vi "DMM_Scan DER Configure and Measure.vi"(0 "Scan Resources Handles In":T2={"DMM Handle"="", "DAQmx Task Out"="", "Relays Status Array"=[], "N Shift Shunt"=1, "Close all Shunts?"=TRUE, "Relays Debounce Time (ms)"=5}, 5 "Scan Configuration":T3[](array[typedef]) {"Resolution in Digits" items=["3 1/2"=3.5, "4 1/2"=4.5, "5 1/2"=5.5, "6 1/2"=6.5, "7 1/2"=7.5]}, 11 "error in":errorcluster) -> (4 "Scan Resources Handles Out":T1={"DMM Handle"="", "DAQmx Task Out"="", "Relays Status Array"=[], "N Shift Shunt"=1, "Close all Shunts?"=TRUE, "Relays Debounce Time (ms)"=5}, 6 "Formatted Measurements":T6[](array[typedef]) {"Switch Time" format="%#_3p"}, 8 "Raw Measurements":T5[](array[typedef]) {"Value" format="%#_8g"}, 10 "Execution Settings":T7[](array[typedef]) {"Function" items=["DC Volts"=1, "AC Volts"=2, "DC Current"=3, "AC Current"=4, "2-Wire Resistance"=5, "4-Wire Resistance"=101, "Frequency"=104, "Period"=105, "AC Volts DC Coupled"=1001, "Diode"=1002, "Waveform Voltage"=1003, "Waveform Current"=1004, "Capacitance"=1005, "Inductance"=1006, "Temperature"=108]; "Absolute\nResolution" format="%#_6p"; "Input Resistance\n(Ohm)" format="%#_6p"; "Range" format="%#_6p"; "Minimum\nFrequency (Hz)" format="%#_6p"; "Aperture\nTime (s)" format="%#_6p"; "Auto Range\nValue" format="%#_6p"; "Settle\nTime (s)" format="%#_6p"}, 14 "Total Scan Time (s)":dbl format="%#.3p", 15 "error out":errorcluster)   [LabVIEW 2021, in "DMM_Scan DAQ Ext RLY.lvlib"]
doc: "Configures an NI-DMM Scan measurement list on the resource provided by the Scan Handle In control according to each given Channel, Function/Range, Digits sub-control. \n\nReturns Formatted Measurements based on Channels and Measurements (string with units), Out of Range, Measurement Time (including configuration, apperture and relay debounce).\n\nReturns Raw Measurements in numeric form to be used and compared in a sequencer.\n \nFor optimization, debugging and reporting, returns Execution Settings and Total Scan Time (s)"
uses:
  DMM_Scan DAQ Ext RLY.lvlib
  Typedefs/Scan configuration.ctl
  <instrlib>/niDMM/nidmm.llb/niDMM Resolution in Digits.ctl
  Typedefs/Measurement values.ctl
  Typedefs/Formatted measurement.ctl
  DMM Mixed Measurements/DMM Mixed Meas Typedefs/DMM Execution Settings.ctl
  Typedefs/Scan Resource Handles In.ctl
  Typedefs/Scan Resource Handles Out.ctl
  DMM Mixed Measurements/DMM Mixed Meas Typedefs/Function Settings.ctl
  Common/Typedefs/Execution Options - Measure.ctl
  DMM Mixed Measurements/DMM_Mixed Measurement.lvlib
  Static Digital State Generation/DAQ_Static Digital State Generation.lvlib
panel:
  # "Inputs"
  # "Outputs"
  # "Channels"
  # "Functions/Range"
  # "Digits"
  # "Channels"
  # "Values"
  # "Units"
  # "Out of R."
  # "Channels"
  # "Measurements"
  # "Out of."
  # "Time"
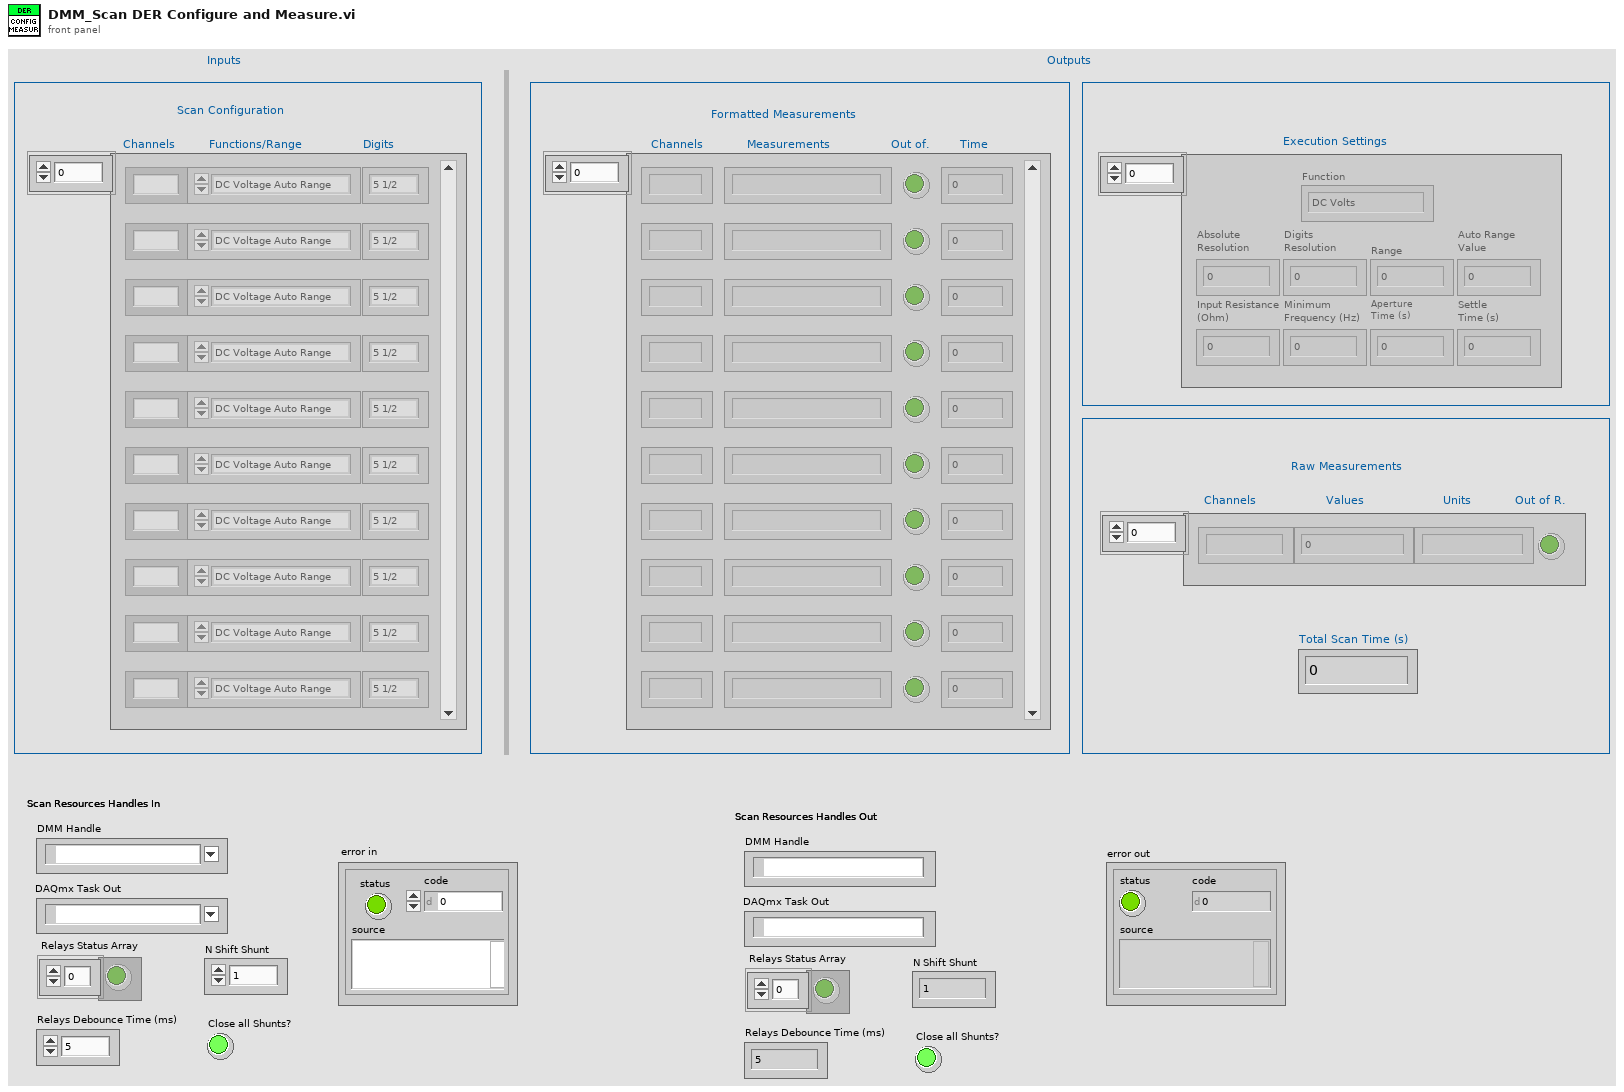
[diagram p1: front panel]
types:
  T1 = typedef "DMM_Scan DAQ Ext RLY.lvlib/Scan Resource Handles Out.ctl" = cluster{"DMM Handle":refnum<k15>, "DAQmx Task Out":refnum<k21>, "Relays Status Array":bool[], "N Shift Shunt":u32, "Close all Shunts?":bool, "Relays Debounce Time (ms)":u32}
  T2 = typedef "DMM_Scan DAQ Ext RLY.lvlib/Scan Resource Handles In.ctl" = cluster{"DMM Handle":refnum<k15>, "DAQmx Task Out":refnum<k21>, "Relays Status Array":bool[], "N Shift Shunt":u32, "Close all Shunts?":bool, "Relays Debounce Time (ms)":u32}
  T3 = typedef "DMM_Scan DAQ Ext RLY.lvlib/Scan configuration.ctl" = cluster{"Channel":string, "Resolution in Digits":T4, "Range and Function":enum16{"DC Voltage Auto Range", "DC 100 mV", "DC 1 V ", "DC 10 V", "DC 100 V", "DC 300 V", " ", "AC Voltage Auto Range", "AC 50 mV", "AC 200 mV", "AC 500 mV", "AC 2 V", "AC 5 V", "AC 20 V", "AC 50 V", "AC 300 V", "  ", "DC Current Auto Range", "DC 1 uA", "DC 10 uA", "DC 100 uA", "DC 1 mA", "DC 10 mA", "DC 20 mA", "DC 100 mA", "DC 200 mA", "DC 1 A", "DC 3 A", "   ", "AC Current Auto Range", "AC 100 uA", "AC 1 mA", "AC 10 mA", "AC 100 mA", "AC 500 mA", "AC 1 A", "AC 3 A", "    ", "Resistance Auto Range", "Res 100 Ohm", "Res 1 kOhm", "Res 10 kOhm", "Res 100 kOhm", "Res 1 MOhm", "Res 10 MOhm", "Res 100 MOhm", "Res 5 GOhm", "     ", "Frequency AC Auto Range", "Freq AC 50 mV", "Freq AC 500 mV", "Freq AC 5 V", "Freq AC 50 V", "Freq AC 300 V", "      ", "Period AC Auto Range", "Period AC 50 mV", "Period AC 500 mV", "Period AC 5 V", "Period AC 50 V", "Period AC 300 V"}}
  T4 = typedef "niDMM Resolution in Digits.ctl" = dbl
  T5 = typedef "DMM_Scan DAQ Ext RLY.lvlib/Measurement values.ctl" = cluster{"Channel":string, "Value":dbl, "Unit":string, "Out of Range":bool}
  T6 = typedef "DMM_Scan DAQ Ext RLY.lvlib/Formatted measurement.ctl" = cluster{"Channel":string, "Switch Time":dbl, "Formatted Measurement":string, "Out of Range":bool}
  T7 = typedef "DMM_Mixed Measurement.lvlib/DMM Execution Settings.ctl" = cluster{"Absolute\nResolution":dbl, "Input Resistance\n(Ohm)":dbl, "Digits\nResolution":dbl, "Range":dbl, "Minimum\nFrequency (Hz)":dbl, "Aperture\nTime (s)":dbl, "Auto Range\nValue":dbl, "Settle\nTime (s)":dbl, "Function":i32}
  T8 = typedef "DMM_Mixed Measurement.lvlib/Function Settings.ctl" = cluster{"Range and Function":enum16{"DC Voltage Auto Range", "DC 100 mV", "DC 1 V ", "DC 10 V", "DC 100 V", "DC 300 V", " ", "AC Voltage Auto Range", "AC 50 mV", "AC 200 mV", "AC 500 mV", "AC 2 V", "AC 5 V", "AC 20 V", "AC 50 V", "AC 300 V", "  ", "DC Current Auto Range", "DC 1 uA", "DC 10 uA", "DC 100 uA", "DC 1 mA", "DC 10 mA", "DC 20 mA", "DC 100 mA", "DC 200 mA", "DC 1 A", "DC 3 A", "   ", "AC Current Auto Range", "AC 100 uA", "AC 1 mA", "AC 10 mA", "AC 100 mA", "AC 500 mA", "AC 1 A", "AC 3 A", "    ", "Resistance Auto Range", "Res 100 Ohm", "Res 1 kOhm", "Res 10 kOhm", "Res 100 kOhm", "Res 1 MOhm", "Res 10 MOhm", "Res 100 MOhm", "Res 5 GOhm", "     ", "Frequency AC Auto Range", "Freq AC 50 mV", "Freq AC 500 mV", "Freq AC 5 V", "Freq AC 50 V", "Freq AC 300 V", "      ", "Period AC Auto Range", "Period AC 50 mV", "Period AC 500 mV", "Period AC 5 V", "Period AC 50 V", "Period AC 300 V"}, "Resolution in Digits":T4}
  T9 = enum16{"DC Voltage Auto Range", "DC 100 mV", "DC 1 V ", "DC 10 V", "DC 100 V", "DC 300 V", " ", "AC Voltage Auto Range", "AC 50 mV", "AC 200 mV", "AC 500 mV", "AC 2 V", "AC 5 V", "AC 20 V", "AC 50 V", "AC 300 V", "  ", "DC Current Auto Range", "DC 1 uA", "DC 10 uA", "DC 100 uA", "DC 1 mA", "DC 10 mA", "DC 20 mA", "DC 100 mA", "DC 200 mA", "DC 1 A", "DC 3 A", "   ", "AC Current Auto Range", "AC 100 uA", "AC 1 mA", "AC 10 mA", "AC 100 mA", "AC 500 mA", "AC 1 A", "AC 3 A", "    ", "Resistance Auto Range", "Res 100 Ohm", "Res 1 kOhm", "Res 10 kOhm", "Res 100 kOhm", "Res 1 MOhm", "Res 10 MOhm", "Res 100 MOhm", "Res 5 GOhm", "     ", "Frequency AC Auto Range", "Freq AC 50 mV", "Freq AC 500 mV", "Freq AC 5 V", "Freq AC 50 V", "Freq AC 300 V", "      ", "Period AC Auto Range", "Period AC 50 mV", "Period AC 500 mV", "Period AC 5 V", "Period AC 50 V", "Period AC 300 V"}
  T10 = typedef "Execution Options - Measure.ctl" = enum16{"Configure & Measure", "Configure only", "Measure only"}
  T11 = cluster{"Range and Function":bool, "Resolution in Digits":bool}
  T12 = typedef "DMM_Mixed Measurement.lvlib/Measurement.ctl" = cluster{"Measured Value":dbl, "Out of Range":bool, "Unit":string, "Measurement":string}
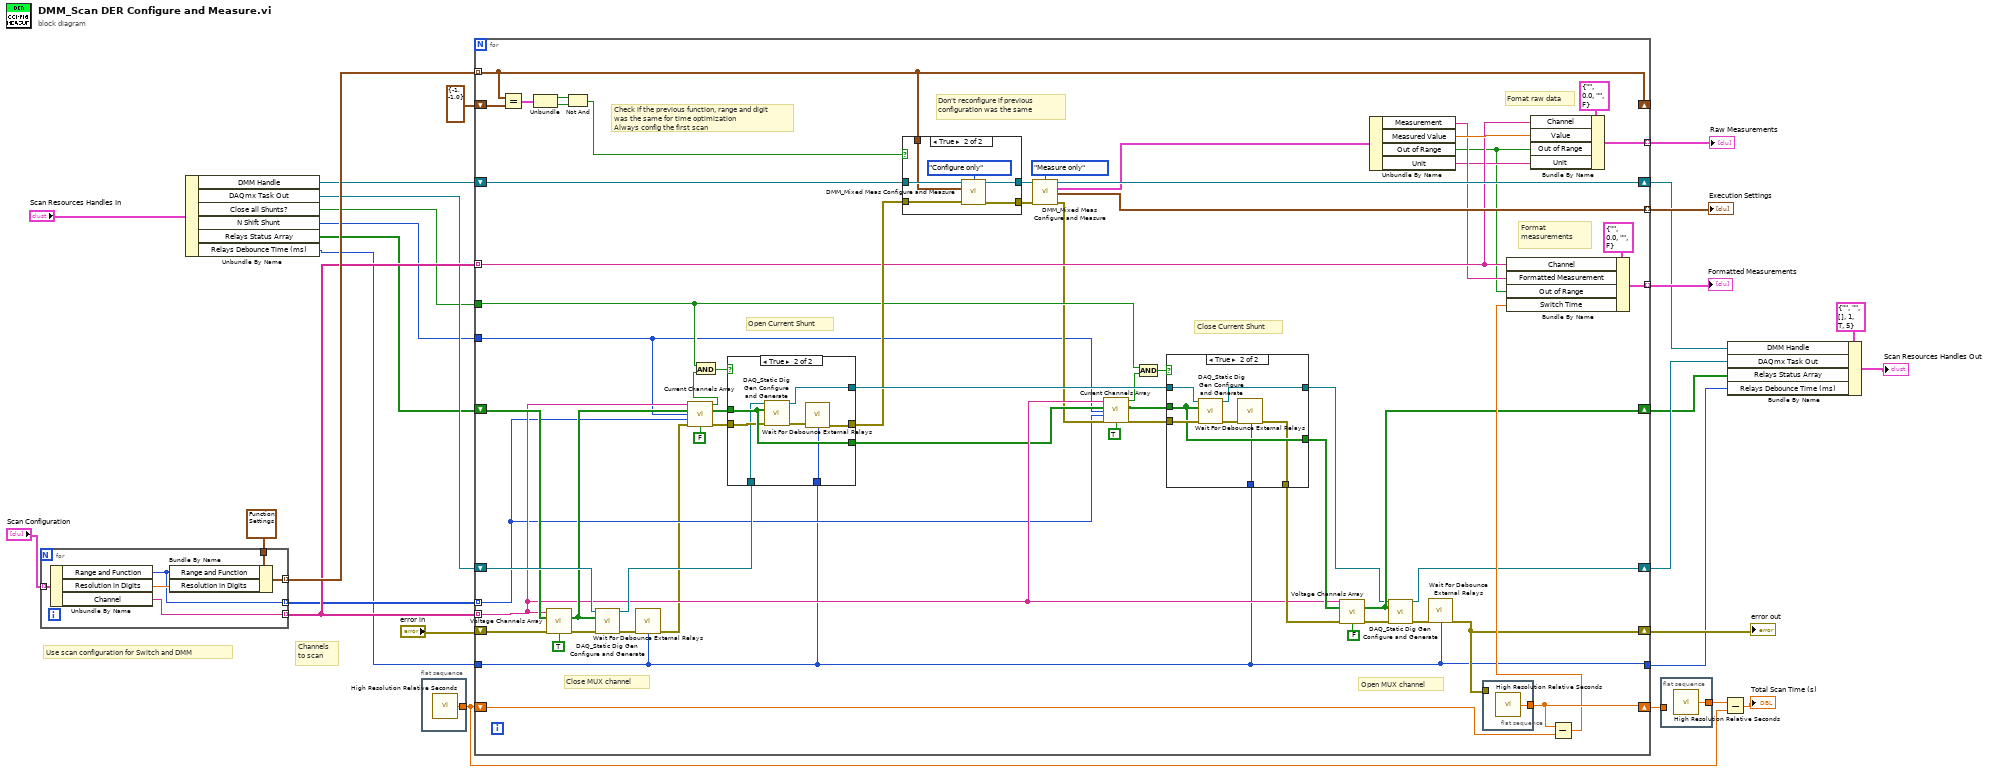
[diagram p0: block diagram]
diagram:
  # "Use scan configuration for Switch and DMM"
  # "Channels\nto scan"
  n1 = for {
    tunnel: "Scan Configuration" -> [w33] mode=indexing
    tunnel: [w34] -> w15 mode=indexing
    tunnel: [w31] -> w28 mode=indexing
    tunnel: T8 {"Range and Function"=enum."DC Voltage Auto Range", "Resolution in Digits"=5.5} ("Function Settings") -> [w30]
    tunnel: [w29] -> w12 mode=indexing
    n2 = Unbundle By Name(w33) -> ("Range and Function"=w29:T9, "Resolution in Digits"=w32:T4, "Channel"=w34:string)
    n3 = Bundle By Name(cluster=w30, "Range and Function"=w29, "Resolution in Digits"=w32) -> (w31:T8)
  }
  n4 = Unbundle By Name("Scan Resources Handles In") -> ("DMM Handle"=w18:refnum<k15>, "DAQmx Task Out"=w11:refnum<k21>, "Close all Shunts?"=w8:bool, "N Shift Shunt"=w7:u32, "Relays Status Array"=w6:bool[], "Relays Debounce Time (ms)"=w5:u32)
  n5 = flat-sequence {
    tunnel: [w35] -> w25
    frame #0 {
      n6 = call <vilib>:"High Resolution Relative Seconds.vi"() -> ("relative seconds"=w35:dbl)
    }
  }
  n7 = for {
    shift-right: [w95] -> w17
    shift-left: w18 -> [w94]
    shift-right: [w57] -> w13
    shift-left: w11 -> [w65]
    shift-right: [w38] -> w14
    shift-left: "error in" -> [w67]
    shift-right: [w97] -> w26
    shift-left: w25 -> [w96]
    tunnel: w28 -> [w82] mode=indexing
    shift-right: [w82] -> _
    shift-left: cluster{i32, dbl} {-1, -1.0} -> [w85]
    tunnel: [w88] -> w19 mode=indexing
    tunnel: w15 -> [w76] mode=indexing
    tunnel: [w78] -> w21 mode=indexing
    tunnel: [w74] -> w20 mode=indexing
    tunnel: w8 -> [w69]
    tunnel: w7 -> [w37]
    tunnel: w15 -> [w52] mode=indexing
    shift-right: [w59] -> w3
    shift-left: w6 -> [w62]
    tunnel: w12 -> [w44] mode=indexing
    tunnel: w5 -> [w36]
    tunnel: [w36] -> w1
    # "Close MUX channel"
    # "Format measurements"
    # "Fomat raw data"
    # "Open MUX channel"
    # "Close Current Shunt"
    # "Open Current Shunt"
    # "Check if the previous function, range and digit was the same for time optimization\nAlways config the first scan"
    # "Don't reconfigure if previous configuration was the same"
    n8 = Equal?(x=w82, y=w85) -> (x = y?=w90:T11)
    n9 = Unbundle(w90) -> ("Range and Function"=w87:bool, "Resolution in Digits"=w86:bool)
    n10 = call "Voltage Channels Array.vi"("Channel 1"=w52, "Relays Array In"=w62, "error in"=w67, "State"=TRUE) -> ("Relay Array out"=w56:bool[], "error out"=w66:errorcluster)  [unwired: 10 in]
    n11 = Not And(1:w86, 2:w87) -> (0:w89:bool)
    n12 = call "DAQ_Static Dig Gen Configure and Generate.vi"("DAQmx Task In"=w65, "Data to Write"=w56, "error in"=w66) -> ("DAQmx Task Out"=w64:refnum<k21>, "error out"=w41:errorcluster)  [unwired: 10 in, 1 out]
    n13 = call "Wait For Debounce External Relays.vi"("error in"=w41, "Wait (ms)"=w36) -> ("error out"=w40:errorcluster)  [unwired: 13 in]
    n14 = call "Current Channels Array.vi"("Channel 1"=w52, "Relays Array In"=w56, "N shift to Min Channel Current"=w37, "Range and Function"=w44, "error in"=w40, "State"=FALSE) -> ("Current Channel?"=w55:bool, "Relay Array out"=w54:bool[], "error out"=w53:errorcluster)  [unwired: 7 in]
    n15 = And(x=w69, y=w55) -> (x .and. y?=w70:bool)
    n16 = case shown="True" w70 {
      tunnel: [w109 w117] -> w84
      tunnel: [w108 w112] -> w83
      tunnel: w36 -> [_ w111]
      tunnel: w54 -> [w110 w116]
      tunnel: [w110 w116] -> w51
      tunnel: w53 -> [w108 w115]
      tunnel: w64 -> [w109 w114]
      frame False {
      }
      frame True {
        n17 = call "DAQ_Static Dig Gen Configure and Generate.vi"("DAQmx Task In"=w114, "Data to Write"=w116, "error in"=w115) -> ("DAQmx Task Out"=w117:refnum<k21>, "error out"=w113:errorcluster)  [unwired: 10 in, 1 out]
        n18 = call "Wait For Debounce External Relays.vi"("error in"=w113, "Wait (ms)"=w111) -> ("error out"=w112:errorcluster)  [unwired: 13 in]
      }
    }
    n19 = case shown="True" w89 {
      tunnel: w94 -> [w119 w125]
      tunnel: [w119 w124] -> w93
      tunnel: [w118 w122] -> w91
      tunnel: w82 -> [_ w120]
      tunnel: w83 -> [w118 w121]
      frame False {
      }
      frame True {
        n20 = call "DMM_Mixed Meas Configure and Measure.vi"("DMM Handle In"=w125, "Execution Option"=Execution_Options_-_Measure."Configure only", "Function Settings"=w120, "error in"=w121) -> ("DMM Handle Out"=w124:refnum<k15>, "error out"=w122:errorcluster)  [unwired: 8 in, 2 out]
      }
    }
    n21 = call "DMM_Mixed Meas Configure and Measure.vi"("DMM Handle In"=w93, "Execution Option"=Execution_Options_-_Measure."Measure only", "error in"=w91) -> ("DMM Handle Out"=w95:refnum<k15>, "Measurement"=w81:T12, "DMM Execution Settings"=w88:T7, "error out"=w50:errorcluster)  [unwired: 9 in]
    n22 = call "Current Channels Array.vi"("Channel 1"=w52, "Relays Array In"=w51, "N shift to Min Channel Current"=w37, "Range and Function"=w44, "error in"=w50, "State"=TRUE) -> ("Current Channel?"=w47:bool, "Relay Array out"=w48:bool[], "error out"=w49:errorcluster)  [unwired: 7 in]
    n23 = And(x=w69, y=w47) -> (x .and. y?=w68:bool)
    n24 = case shown="True" w68 {
      tunnel: w84 -> [w100 w107]
      tunnel: [w100 w106] -> w58
      tunnel: [w99 w101] -> w60
      tunnel: w36 -> [_ w102]
      tunnel: w49 -> [w99 w105]
      tunnel: [w98 w104] -> w61
      tunnel: w48 -> [w98 w104]
      frame False {
      }
      frame True {
        n25 = call "DAQ_Static Dig Gen Configure and Generate.vi"("DAQmx Task In"=w107, "Data to Write"=w104, "error in"=w105) -> ("DAQmx Task Out"=w106:refnum<k21>, "error out"=w103:errorcluster)  [unwired: 10 in, 1 out]
        n26 = call "Wait For Debounce External Relays.vi"("error in"=w103, "Wait (ms)"=w102) -> ("error out"=w101:errorcluster)  [unwired: 13 in]
      }
    }
    n27 = call "Voltage Channels Array.vi"("Channel 1"=w52, "Relays Array In"=w61, "error in"=w60, "State"=FALSE) -> ("Relay Array out"=w59:bool[], "error out"=w63:errorcluster)  [unwired: 10 in]
    n28 = Unbundle By Name(w81) -> ("Measurement"=w75:string, "Measured Value"=w79:dbl, "Out of Range"=w72:bool, "Unit"=w73:string)
    n29 = call "DAQ_Static Dig Gen Configure and Generate.vi"("DAQmx Task In"=w58, "Data to Write"=w59, "error in"=w63) -> ("DAQmx Task Out"=w57:refnum<k21>, "error out"=w39:errorcluster)  [unwired: 10 in, 1 out]
    n30 = call "Wait For Debounce External Relays.vi"("error in"=w39, "Wait (ms)"=w36) -> ("error out"=w38:errorcluster)  [unwired: 13 in]
    n31 = flat-sequence {
      tunnel: [w126] -> w97
      tunnel: w38 -> [_]
      frame #0 {
        n32 = call <vilib>:"High Resolution Relative Seconds.vi"() -> ("relative seconds"=w126:dbl)
      }
    }
    n33 = Bundle By Name(cluster=T5 {"Channel"="", "Value"=0.0, "Unit"="", "Out of Range"=FALSE} ("Measurements"), "Channel"=w76, "Value"=w79, "Out of Range"=w72, "Unit"=w73) -> (w78:T5)
    n34 = Subtract(x=w97, y=w96) -> (x-y=w71:dbl)
    n35 = Bundle By Name(cluster=T6 {"Channel"="", "Switch Time"=0.0, "Formatted Measurement"="", "Out of Range"=FALSE} ("Measurements"), "Channel"=w76, "Formatted Measurement"=w75, "Out of Range"=w72, "Switch Time"=w71) -> (w74:T6)
  }
  "error out" <- w14
  "Raw Measurements" <- w21
  "Formatted Measurements" <- w20
  "Execution Settings" <- w19
  n36 = flat-sequence {
    tunnel: [w127] -> w24
    tunnel: w26 -> [_]
    frame #0 {
      n37 = call <vilib>:"High Resolution Relative Seconds.vi"() -> ("relative seconds"=w127:dbl)
    }
  }
  n38 = Subtract(x=w24, y=w25) -> (x-y=→"Total Scan Time (s)":dbl)
  n39 = Bundle By Name(cluster=T1 {"DMM Handle"="", "DAQmx Task Out"="", "Relays Status Array"=[], "N Shift Shunt"=1, "Close all Shunts?"=TRUE, "Relays Debounce Time (ms)"=5} ("Scan Resources Handles Out"), "DMM Handle"=w17, "DAQmx Task Out"=w13, "Relays Status Array"=w3, "Relays Debounce Time (ms)"=w1) -> (→"Scan Resources Handles Out":T1)
